vi "Drivetrain.vi"() -> ()   [LabVIEW 2012]
uses:
  <vilib>/Rock Robotics/WPI/Solenoid/WPI_SolenoidValue.ctl
  Robot Global Data.vi
  <vilib>/addons/control/pid/pid.llb/PID (DBL).vi
  <vilib>/Rock Robotics/WPI/RobotDrive/WPI_RobotDriveGetSetRefNum.vi
  <vilib>/addons/control/pid/NI_PID_pid.lvlib
panel:
  in  "PID gains":T1={"proportional gain (Kc)"=20.0, "integral time (Ti, min)"=0.008, "derivative time (Td, min)"=0.001} {"derivative time (Td, min)" format="%.3f"; "integral time (Ti, min)" format="%.3f"; "proportional gain (Kc)" format="%.3f"}
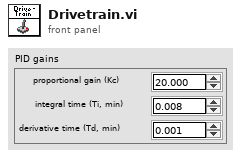
[diagram p1: front panel]
types:
  T1 = cluster{"proportional gain (Kc)":dbl, "integral time (Ti, min)":dbl, "derivative time (Td, min)":dbl}
  T2 = typedef "WPI_SolenoidValue.ctl" = enum16{"Off", "On", "Forward", "Reverse"}
  T3 = typedef "WPI_RelayDevRef.ctl" = cluster{"DevStatus":errorcluster, "Relay Channel":T4, "Digital Module":T5, "Relay Direction":T6}
  T4 = typedef "FPGA_DIORelayChannel.ctl" = enum8{"Relay 1", "Relay 2", "Relay 3", "Relay 4", "Relay 5", "Relay 6", "Relay 7", "Relay 8", "Invalid"}
  T5 = typedef "FPGA_TypedefDigitalModule.ctl" = enum16{"Digital Module 1", "Digital Module 2"}
  T6 = typedef "WPI_RelayDirection.ctl" = enum16{"Both directions", "Forward only", "Reverse only"}
  T7 = typedef "WPI_RobotDriveDevRef.ctl" = cluster{"DevStatus":errorcluster, "Motors[]":T8[], "Square Inputs":bool, "Max Output":dbl, "Isochronous":bool}
  T8 = typedef "WPI_MotorControlDeviceRef.ctl" = cluster{"DeviceStatus":errorcluster, "Type":enum16{"PWM", "CAN"}, "PWM":cluster{"Digital Module":T5, "PWM Channel":T9, "DeadBand":T10}, "CAN":cluster{"Device Number":u8, "Control Mode":T11, "Semaphore":T12, "Max Vout":dbl}, "Invert":bool, "TransformRef":T13, "InvTransformRef":T13}
  T9 = typedef "FPGA_DIOPWMChannel.ctl" = enum8{"PWM 1", "PWM 2", "PWM 3", "PWM 4", "PWM 5", "PWM 6", "PWM 7", "PWM 8", "PWM 9", "PWM 10", "Invalid"}
  T10 = typedef "WPI_PWMDeadband.ctl" = cluster{"Name":string, "maxPositivePwm":i32, "minPositivePwm":i32, "centerPwm":i32, "maxNegativePwm":i32, "minNegativePwm":i32, "angularRange":u16}
  T11 = typedef "WPI_CANJaguar_ControlMode.ctl" = enum8{"Percent VBus", "Current", "Speed", "Position", "Voltage"}
  T12 = typedef "Semaphore RefNum" = refnum<k1>
  T13 = typedef "WPI_PWMTransform_ConPane.ctl" = refnum<vi>
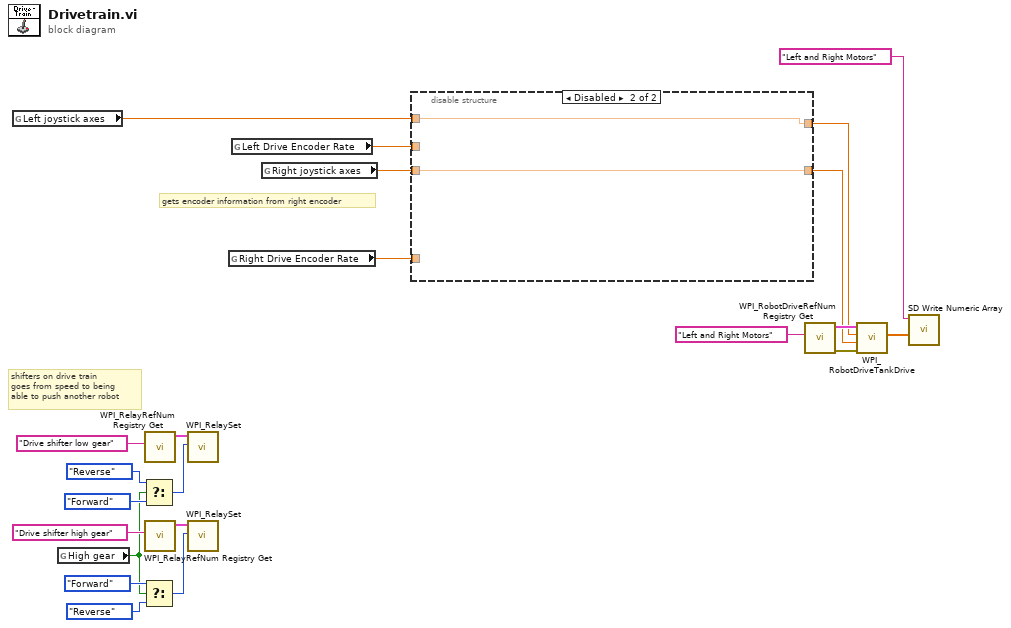
[diagram p0: block diagram]
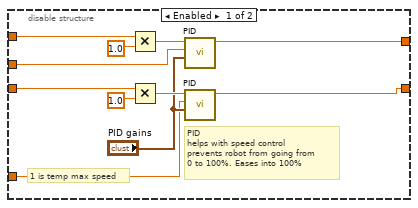
[diagram p2: hidden frame]
diagram:
  # "shifters on drive train\ngoes from speed to being\nable to push another robot"
  # "gets encoder information from right encoder"
  n1 = global read "Robot Global Data.vi" "Left joystick axes"() -> (w13:dbl)
  n2 = global read "Robot Global Data.vi" "High gear"() -> (w1:bool)
  n3 = Select(t=WPI_SolenoidValue."Reverse" ("Value"), s=w1, f=WPI_SolenoidValue."Forward" ("Value")) -> (s? t:f=w4:T2)
  n4 = Select(t=WPI_SolenoidValue."Forward" ("Value"), s=w1, f=WPI_SolenoidValue."Reverse" ("Value")) -> (s? t:f=w5:T2)
  n5 = call <vilib>:"WPI_RelayRefNum Registry Get.vi"("refnum name"="Drive shifter low gear") -> ("RelayDevRef"=w2:T3)  [unwired: 9 in, 1 out]
  n6 = call <vilib>:"WPI_RelayRefNum Registry Get.vi"("refnum name"="Drive shifter high gear") -> ("RelayDevRef"=w3:T3)  [unwired: 9 in, 1 out]
  n7 = call <vilib>:"WPI_RelaySet.vi"("RelayValue"=w4, "RelayDevRef"=w2) -> ()  [unwired: 8 in, 2 out]
  n8 = call <vilib>:"WPI_RelaySet.vi"("RelayValue"=w5, "RelayDevRef"=w3) -> ()  [unwired: 8 in, 2 out]
  n9 = global read "Robot Global Data.vi" "Right Drive Encoder Rate"() -> (w20:dbl)
  n10 = global read "Robot Global Data.vi" "Left Drive Encoder Rate"() -> (w19:dbl)
  n11 = global read "Robot Global Data.vi" "Right joystick axes"() -> (w12:dbl)
  n12 = disable-structure shown="Disabled" {
    disable-tunnel: w13 -> [w32 w35]
    disable-tunnel: [w30 w35] -> w16
    disable-tunnel: w19 -> [w29 _]
    disable-tunnel: [w25 w34] -> w15
    disable-tunnel: w20 -> [w24 _]
    disable-tunnel: w12 -> [w23 w34]
    frame Enabled {
      # "1 is temp max speed"
      # "PID\nhelps with speed control \nprevents robot from going from\n0 to 100%. Eases into 100%"
      n13 = Multiply(x=w32, y=1.0) -> (x*y=w31:dbl)
      n14 = Multiply(x=w23, y=1.0) -> (x*y=w27:dbl)
      n15 = call-poly <vilib>:"PID.vi"("PID gains"="PID gains", "process variable"=w29, "setpoint"=w31) -> ("output"=w30:dbl)  [unwired: 7 in, 1 out]
      n16 = call-poly <vilib>:"PID.vi"("PID gains"="PID gains", "process variable"=w24, "setpoint"=w27) -> ("output"=w25:dbl)  [unwired: 7 in, 1 out]
    }
    frame Disabled {
    }
  }
  n17 = call <vilib>:"WPI_RobotDriveRefNum Registry Get.vi"("refnum name"="Left and Right Motors") -> ("error out"=w14:errorcluster, "RobotDriveDevRef"=w22:T7)  [unwired: 1 in, 8 out]
  n18 = call <vilib>:"WPI_RobotDriveTankDrive.vi"("error in (no error)"=w14, "Right axis value"=w15, "Left axis value"=w16, "RobotDriveDevRef"=w22) -> ("Motor Values"=w18:dbl[])  [unwired: 5 in, 2 out]
  n19 = call <vilib>:"SD Write Numeric Array.vi"("Numeric Array"=w18, "Name"="Left and Right Motors") -> ()  [unwired: 8 in, 2 out]
